vi "Current_Measurement.vi"() -> ()   [LabVIEW 2011]
uses:
  <vilib>/Utility/file.llb/Read From Spreadsheet File (DBL).vi
panel:
  in  "run":bool
  in  "stop":bool
  in  "Slide":i32(slide) scale=0.0..22500.0
  out "Waveform Graph":dbl[][](graph)
  out "Values in .csv file":string[][](array[string])
  in  "File Path for .csv file with current values":path
  in  "Enable Measurement":bool
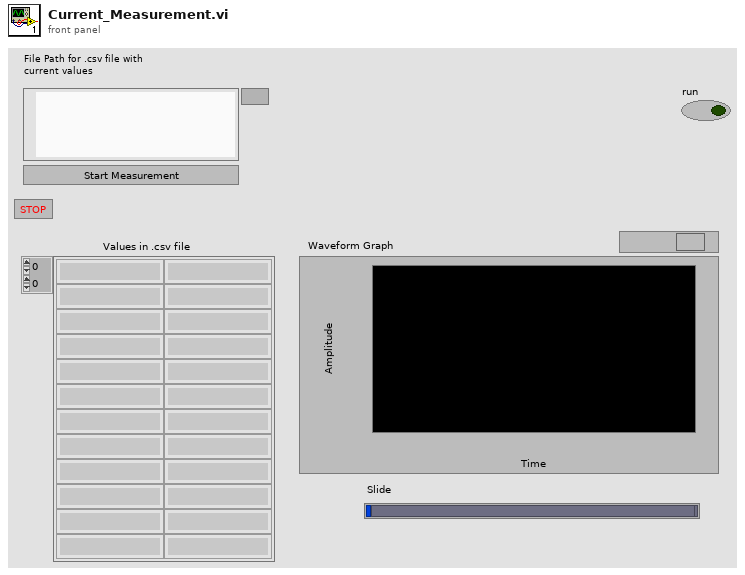
[diagram p1: front panel]
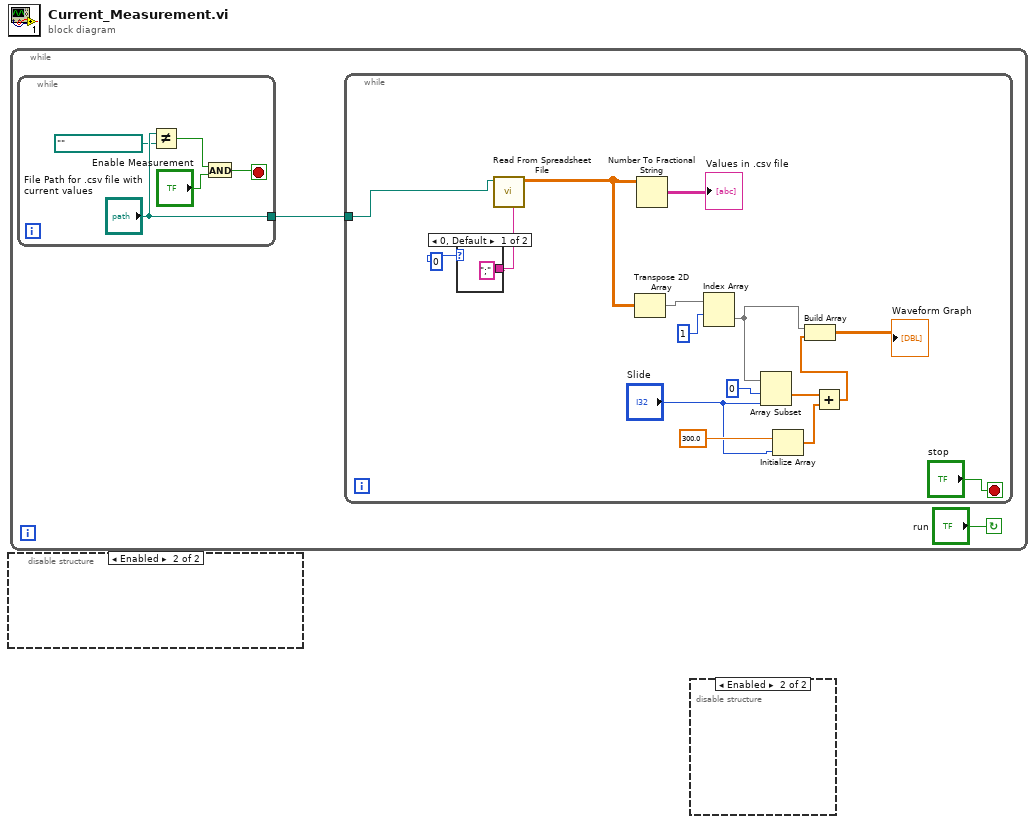
[diagram p0: block diagram]
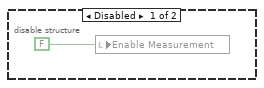
[diagram p2: hidden frame]
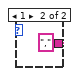
[diagram p3: hidden frame]
diagram:
  n1 = disable-structure shown="Enabled" {
    frame Disabled {
      n2 = local write "Enable Measurement"(FALSE ("Enable Measurement")) -> ()
    }
    frame Enabled {
    }
  }
  n3 = while {
    stop <- "run" continue-if-true
    n4 = while {
      tunnel: ["File Path for .csv file with current values"] -> w3
      stop <- w4 stop-if-true
      n5 = Not Equal?(x="File Path for .csv file with current values", y=path "") -> (x != y?=w5:bool)
      n6 = And(x=w5, y="Enable Measurement") -> (x .and. y?=w4:bool)
    }
    n7 = while {
      tunnel: w3 -> [w11]
      stop <- "stop" stop-if-true
      n8 = case shown="0, Default" 0 {
        tunnel: [";" ("delimiter (\\t)") ","] -> w22
        frame 0, Default {
        }
        frame 1 {
        }
      }
      n9 = call-poly <vilib>:"Read From Spreadsheet File.vi"("delimiter (\\t)"=w22, "file path (dialog if empty)"=w11) -> ("all rows"=w21:dbl[][])  [unwired: 5 in, 4 out]
      n10 = Transpose 2D Array(2D array=w21) -> (transposed array=w16:dbl[][])
      n11 = Number To Fractional String(number=w21) -> (F-format string=→"Values in .csv file":string[][])  [unwired: 3 in]
      n12 = Index Array(array=w16, index (row)=1 ("length")) -> (element=w15:dbl[])  [unwired: 1 in]
      n13 = Array Subset(array=w15, index=0, length="Slide") -> (w19:dbl[])
      n14 = Initialize Array(300.0 ("element"), "Slide") -> (w12:dbl[])
      n15 = Add(x=w19, y=w12) -> (x+y=w18:dbl[])
      n16 = Build Array(w15, w18) -> (→"Waveform Graph":dbl[][])
    }
  }
  n17 = disable-structure shown="Enabled" {
    frame Disabled {
    }
    frame Enabled {
    }
  }
